vi "Copy.vi"(11 "TypedCircularBuffer in":refnum<class "RotateCircularBuffer.lvclass">) -> (2 "Copied Buffer":T1[](array[typedef]), 3 "TypedCircularBuffer out":refnum<class "RotateCircularBuffer.lvclass">)   [LabVIEW 2024, in "RotateCircularBuffer.lvclass"]
uses:
  RotateCircularBuffer.lvclass
  Type.ctl
  RotateCircularBuffer.lvclass/RotateCircularBuffer.ctl
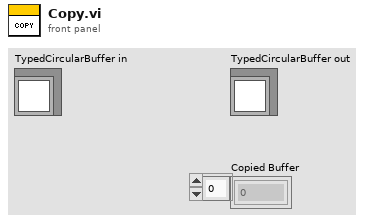
[diagram p1: front panel]
types:
  T1 = typedef "RotateCircularBuffer.lvclass/Type.ctl" = u8
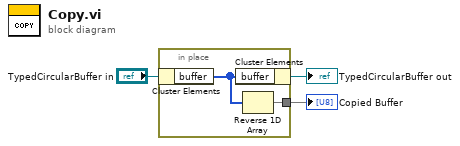
[diagram p0: block diagram]
diagram:
  n1 = in-place {
    in-place-border: [w4] -> w1
    n2 = in-place-cluster #1("TypedCircularBuffer in") -> ("buffer"=w5:T1[])
    n3 = in-place-cluster #1("buffer"=w5) -> (→"TypedCircularBuffer out":refnum<class "RotateCircularBuffer.lvclass">)
    n4 = Reverse 1D Array(array=w5) -> (reversed array=w4:T1[])
  }
  "Copied Buffer" <- w1
